vi "Prepare CLI Arguments.vi"(8 "error in":errorcluster, 10 "Marker Mapping":map{string, string}(c390)) -> (0 "error out":errorcluster, 2 "Arguments":map{string, string}(c390), 3 "application name":string)   [LabVIEW 2021, in "Bananas.lvlib"]
uses:
  Bananas/Bananas.lvlib
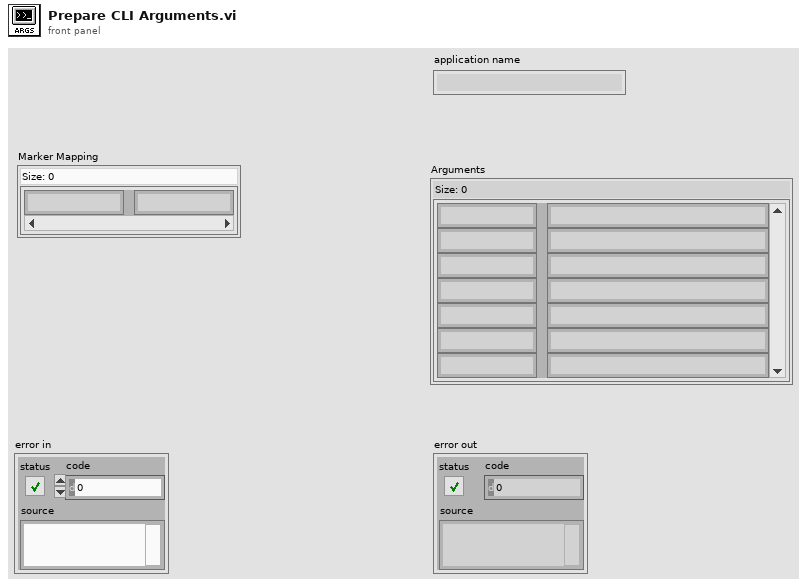
[diagram p1: front panel]
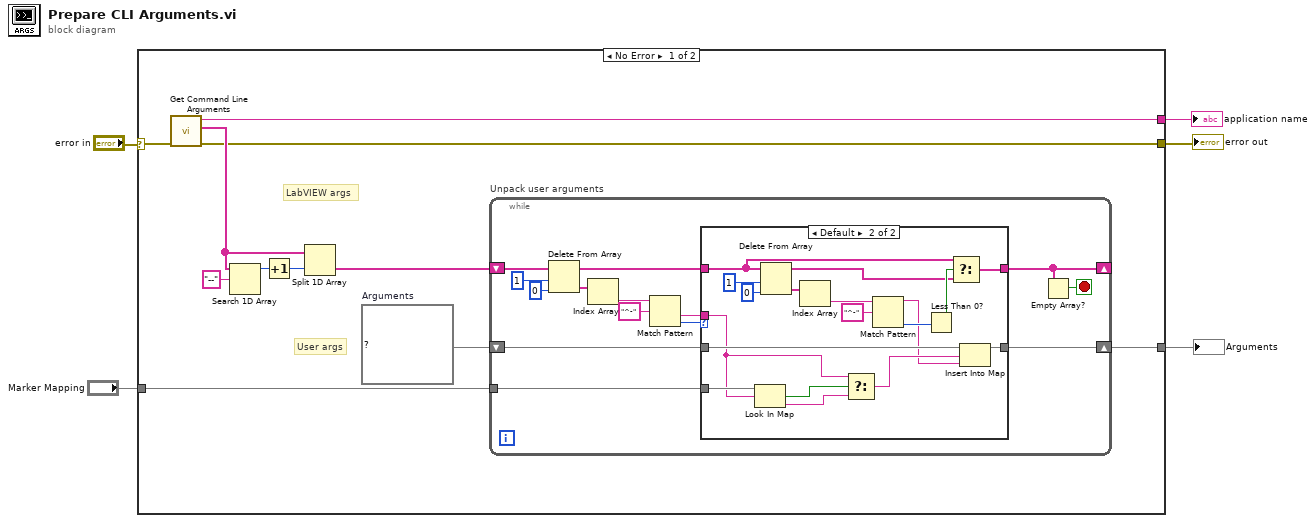
[diagram p0: block diagram]
diagram:
  n1 = case shown="No Error" "error in" {
    selector: "error in" -> [w7 w51]
    tunnel: [w11 _] -> w5
    tunnel: "Marker Mapping" -> [w9 _]
    tunnel: [w8 _] -> w3
    tunnel: [w6 w51] -> w2
    frame No Error {
      w12 = map{string, string} {}  # Arguments
      # "User args"
      # "LabVIEW args"
      n2 = call <vilib>:"Get Command Line Arguments.vi"("error in (no error)"=w7) -> ("error out"=w6:errorcluster, "arguments"=w15:string[], "application name"=w8:string)  [unwired: 8 in]
      n3 = Search 1D Array(1D array=w15, element="--") -> (index of element=w14:i32)  [unwired: 1 in]
      n4 = Increment(x=w14) -> (x+1=w10:i32)
      n5 = Split 1D Array(array=w15, index=w10) -> (second subarray=w13:string[])  [unwired: 1 out]
      n6 = while "Unpack user arguments" {
        shift-right: [w24] -> _
        shift-left: w13 -> [w29]
        shift-right: [w23] -> w11
        shift-left: w12 -> [w22]
        tunnel: w9 -> [w18]
        stop <- w30 stop-if-true
        n7 = Delete From Array(array=w29, length=1, index=0) -> (deleted portion=w26:string[], array with subset deleted=w25:string[])
        n8 = Index Array(array=w26) -> (element=w17:string)  [unwired: 1 in]
        n9 = Match Pattern(string=w17, regular expression="^-") -> (after substring=w19:string, offset past match=w21:i32)  [unwired: 1 in, 2 out]
        n10 = case shown="Default" w21 {
          tunnel: w25 -> [w32 w41]
          tunnel: [w32 w39] -> w24
          tunnel: [w31 w47] -> w23
          tunnel: w22 -> [w31 w44]
          tunnel: w19 -> [_ w34]
          tunnel: w18 -> [_ w38]
          frame -1 {
          }
          frame Default {
            n11 = Look In Map(map=w38, key=w34) -> (key not found?=w37:bool, value=w36:string)  [unwired: 1 in]
            n12 = Delete From Array(array=w41, length=1, index=0) -> (deleted portion=w50:string[], array with subset deleted=w40:string[])
            n13 = Index Array(array=w50) -> (element=w45:string)  [unwired: 1 in]
            n14 = Select(t=w34, s=w37, f=w36) -> (s? t:f=w35:string)
            n15 = Match Pattern(string=w45, regular expression="^-") -> (before substring=w33:string, offset past match=w42:i32)  [unwired: 1 in, 2 out]
            n16 = Less Than 0?(x=w42) -> (x < 0?=w43:bool)
            n17 = Select(t=w41, s=w43, f=w40) -> (s? t:f=w39:string[])
            n18 = Insert Into Map(map in=w44, key=w35, value=w33) -> (map out=w47:map{string, string})  [unwired: 2 out]
          }
        }
        n19 = Empty Array?(array=w24) -> (empty?=w30:bool)
      }
    }
    frame Error {
    }
  }
  "Arguments" <- w5
  "application name" <- w3
  "error out" <- w2
